vi "Interactive voltage setting on slow analog output.vi"() -> ()   [LabVIEW 2010]
doc: "This example shows how to set analog voltage on slow analog Red Pitaya outputs using LabVIEW slider. Slow analog outputs on Red Pitaya are in range from 0 to 1.8 Volts."
uses:
  RedPitaya.lvlib
panel:
  in  "Pin #":u16(ring)=3 items=["AOUT0", "AOUT1", "AOUT2", "AOUT3"]
  in  "Set Analog Voltage":dbl(slide) scale=0.0..1.8
  in  "IP address":string="192.168.4.129"
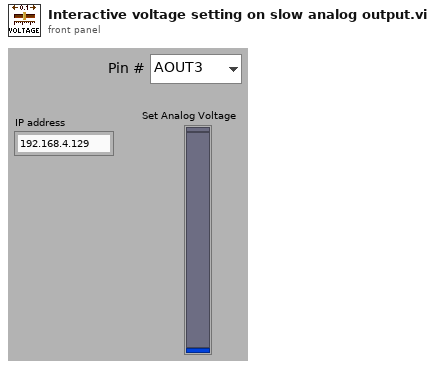
[diagram p1: front panel]
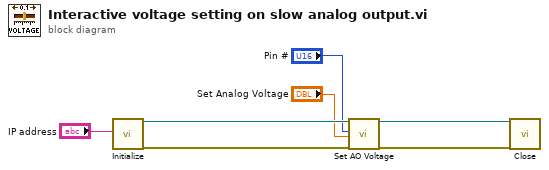
[diagram p0: block diagram]
diagram:
  n1 = call "Initialize.vi"("IP address"="IP address") -> ("RedPitaya connection out"=w6:refnum<k5>, "error out"=w5:errorcluster)  [unwired: 17 in]
  n2 = call "Set AO Voltage.vi"("RedPitaya connection in"=w6, "Pin #"="Pin #", "Analog Voltage Value"="Set Analog Voltage", "error in"=w5) -> ("RedPitaya connection out"=w3:refnum<k5>, "error out"=w4:errorcluster)  [unwired: 14 in]
  n3 = call "Close.vi"("RedPitaya connection in"=w3, "error in"=w4) -> ()  [unwired: 17 in, 1 out]
